vi "Check_Traverse_move.vi"(0 "Current position":sgl[](array[numeric])=[0.0, 0.0, 0.0] format="%.2f", 1 "Traverse Name":string, 2 "Full Check":bool, 5 "New Position":sgl[](array[numeric])=[0.0, 0.0, 0.0] format="%.2f", 7 "Model       Roll      Pitch       Yaw (deg)":sgl[](array[numeric]) format="%#.2f", 9 "Probe Volume":T1=[{"Max"=15.0, "Min"=-15.0}, {"Max"=250.0, "Min"=0.0}, {"Max"=15.0, "Min"=-15.0}] {"Min" format="%#.1f"; "Max" format="%#.1f"}, 11 "Entire Space":T1=[{"Max"=15001.0, "Min"=12000.0}, {"Max"=1000.0, "Min"=-1000.0}, {"Max"=700.0, "Min"=0.0}] {"Min" format="%#.1f"; "Max" format="%#.1f"}, 12 "Exclude Array":T2[](array[typedef])=[{"Sizes"=[{"Max"=15000.0, "Min"=0.0}, {"Max"=1000.0, "Min"=-1000.0}, {"Max"=300.0, "Min"=0.0}], "Name"="Roughness Elements", "Exclude Type"=enum."Allow only vertical moves"}, {"Sizes"=[{"Max"=17000.0, "Min"=16000.0}, {"Max"=200.0, "Min"=-200.0}, {"Max"=-50.0, "Min"=-250.0}], "Name"="B204", "Exclude Type"=enum."Exclude completely"}] {"Sizes"."Min" format="%#.1f"; "Sizes"."Max" format="%#.1f"}, 13 "Probe Support":T1=[{"Max"=15001.0, "Min"=12000.0}, {"Max"=1000.0, "Min"=-1000.0}, {"Max"=700.0, "Min"=0.0}] {"Min" format="%#.1f"; "Max" format="%#.1f"}) -> (6 "Position At Crash":dbl[](array[numeric]) format="%.2f", 10 "Steps":sgl[][](array[numeric]) format="%.2f", 15 "Error Comments":string)   [LabVIEW 2020]
uses:
  Box_size.ctl
  Exclude_cluster.ctl
  Exclusion_type.ctl
panel:
  # "X                Y                   Z"
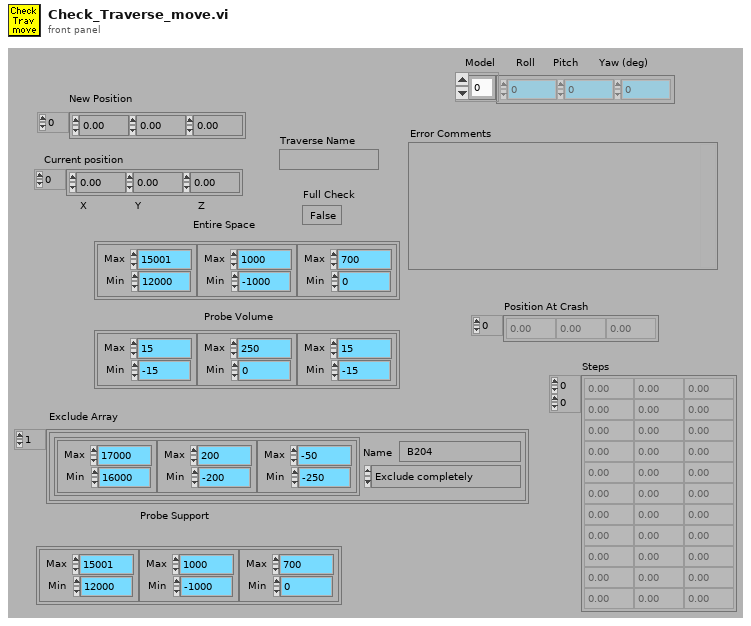
[diagram p1: front panel]
types:
  T1 = typedef "Box_size.ctl" = cluster{"Max":sgl, "Min":sgl}[]
  T2 = typedef "Exclude_cluster.ctl" = cluster{"Sizes":T1, "Name":string, "Exclude Type":T3}
  T3 = typedef "Exclusion_type.ctl" = enum16{"Exclude completely", "Allow only vertical moves"}
  T4 = enum16{"To Traverse Coordinates", "To User Coordinates"}
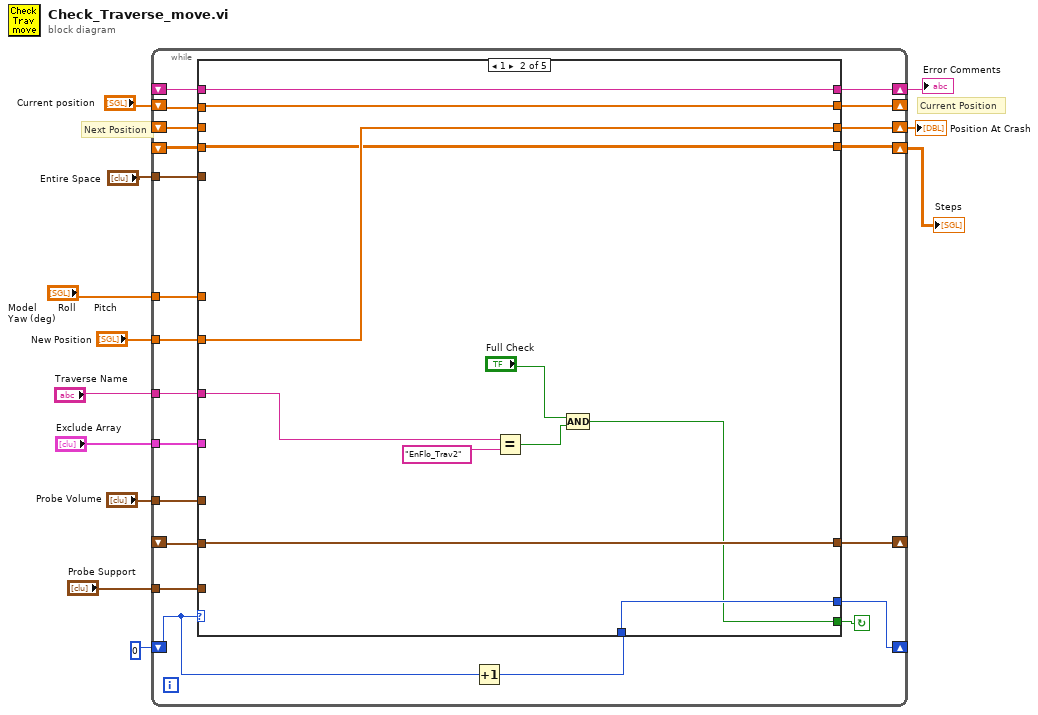
[diagram p0: block diagram]
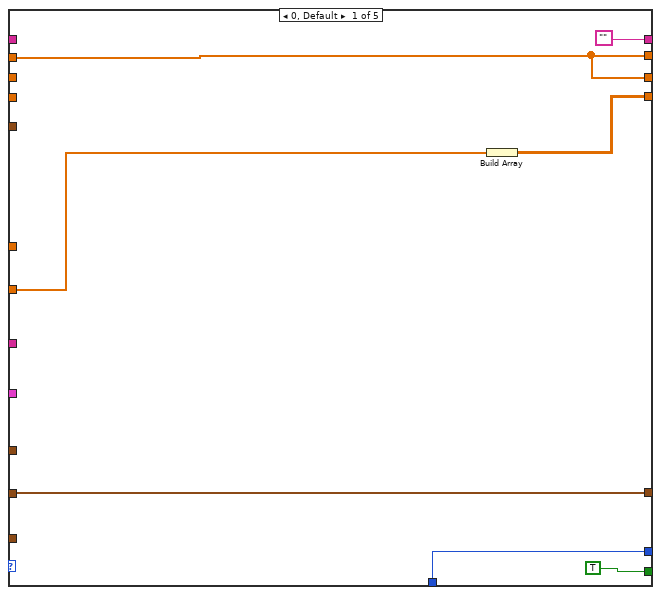
[diagram p2: hidden frame]
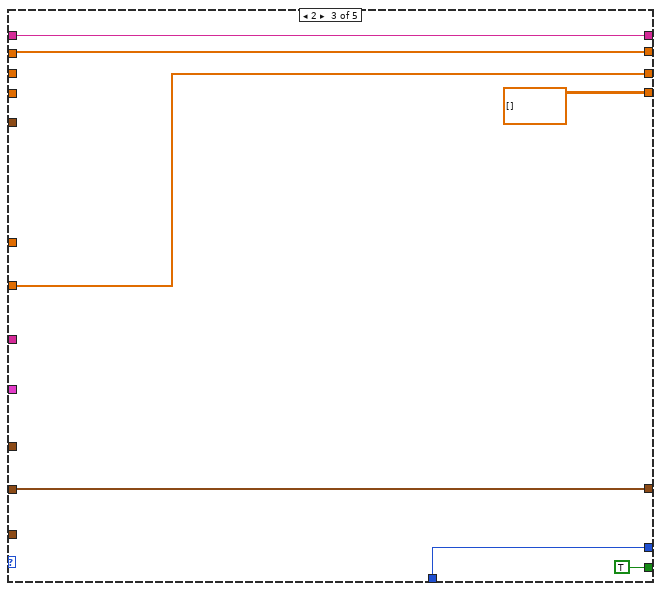
[diagram p3: hidden frame]
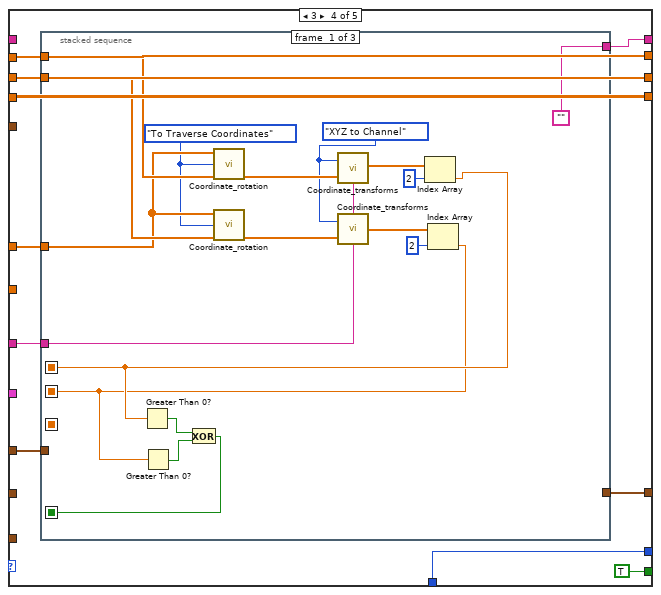
[diagram p4: hidden frame]
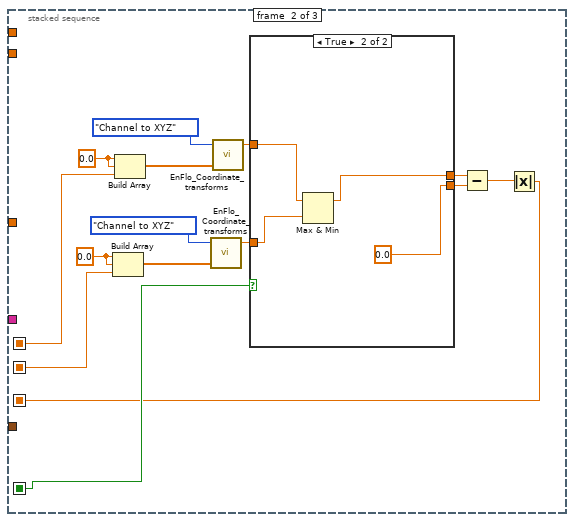
[diagram p5: hidden frame]
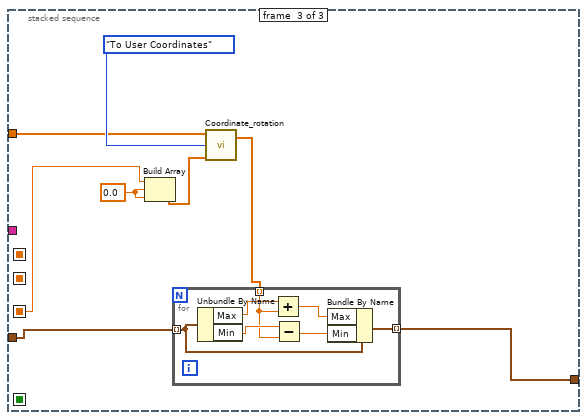
[diagram p7: hidden frame]
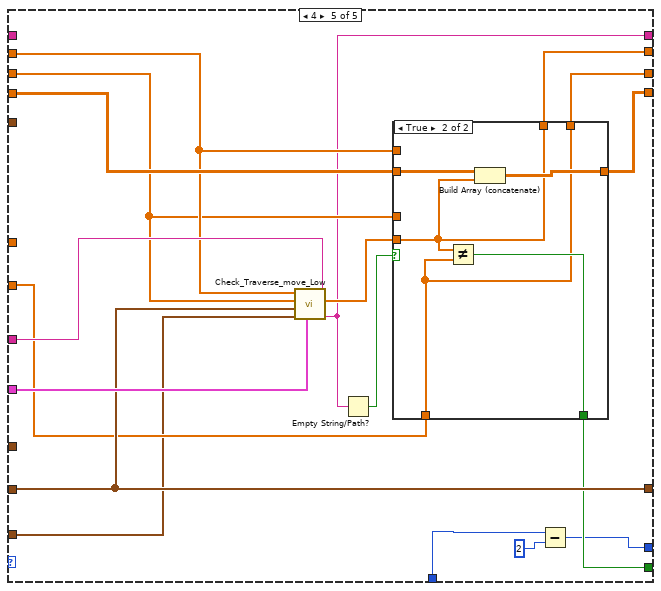
[diagram p8: hidden frame]
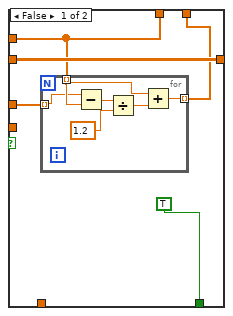
[diagram p9: hidden frame]
diagram:
  # "Current Position"
  # "Next Position"
  n1 = while {
    shift-left: _ -> [w15]
    shift-right: [w14] -> w3
    tunnel: "Probe Volume" -> [w16]
    shift-left: _ -> [w18]
    shift-right: [w17] -> _
    tunnel: "Model       Roll      Pitch       Yaw (deg)" -> [w19]
    tunnel: "New Position" -> [w20]
    shift-left: _ -> [w22]
    shift-right: [w23] -> w7
    shift-left: 0 -> [w26]
    shift-right: [w25] -> _
    tunnel: "Traverse Name" -> [w27]
    tunnel: "Entire Space" -> [w28]
    tunnel: "Exclude Array" -> [w29]
    shift-left: _ -> [w21]
    shift-right: [w31] -> w5
    shift-left: "Current position" -> [w33]
    shift-right: [w32] -> _
    tunnel: "Probe Support" -> [w13]
    stop <- w30 continue-if-true
    n2 = Increment(x=w26) -> (x+1=w24:i32)
    n3 = case shown="1" w26 {
      tunnel: w33 -> [w34 w50 w57 w65 w126]
      tunnel: [w34 w50 w57 w65 w131] -> w32
      tunnel: [w34 w43 w54 w64 w130] -> w31
      tunnel: [TRUE ("Box Inside") w45 TRUE ("Box Inside") TRUE ("Box Inside") w133] -> w30
      tunnel: w18 -> [w40 w49 w56 _ w138]
      tunnel: w29 -> [_ _ _ _ w140]
      tunnel: w28 -> [_ _ _ _ _]
      tunnel: w27 -> [_ w46 _ w62 w139]
      tunnel: [w36 w48 w55 w60 w128] -> w25
      tunnel: w24 -> [w36 w48 w55 w60 w127]
      tunnel: ["" w51 w58 w68 w123] -> w23
      tunnel: w22 -> [_ w51 w58 _ _]
      tunnel: w21 -> [_ _ _ w64 w125]
      tunnel: w20 -> [w39 w43 w54 _ w134]
      tunnel: w19 -> [_ _ _ w63 _]
      tunnel: [w40 w49 w56 w66 w138] -> w17
      tunnel: w16 -> [_ _ _ w61 _]
      tunnel: w15 -> [_ w42 _ w59 w137]
      tunnel: [w38 w42 dbl[][] [] w59 w136] -> w14
      tunnel: w13 -> [_ _ _ _ w124]
      frame 0, Default {
        n4 = Build Array(w39) -> (w38:sgl[][])
      }
      frame 1 {
        n5 = Equal?(x=w46, y="EnFlo_Trav2") -> (x = y?=w41:bool)
        n6 = Compound Arithmetic op=AND("Full Check", w41) -> (w45:bool)
      }
      frame 2 {
      }
      frame 3 {
        n7 = stacked-sequence {
          seq-local: [w71 _ _] -> [_ w101 _]
          seq-local: [w70 _ _] -> [_ w100 _]
          seq-local: [w69 _ _] -> [_ w91 _]
          seq-local: [_ w87 _] -> [_ _ w110]
          tunnel: ["" _ _] -> w68
          tunnel: [_ _ w114] -> w66
          tunnel: w65 -> [w84 _ _]
          tunnel: w64 -> [w82 _ _]
          tunnel: w63 -> [w81 _ w108]
          tunnel: w62 -> [w80 _ _]
          tunnel: w61 -> [_ _ w115]
          frame #0 {
            w78 = enum16{"XYZ to Channel", "Channel to XYZ"}."XYZ to Channel" ("Mode")
            w79 = T4."To Traverse Coordinates" ("Mode")
            n8 = call "Coordinate_rotation.vi"("Roll-Pitch-Yaw"=w81, "Input Position"=w84, "Mode"=w79) -> ("Output Position"=w85:sgl[])  [unwired: 2 in, 1 out]
            n9 = call "Coordinate_rotation.vi"("Roll-Pitch-Yaw"=w81, "Input Position"=w82, "Mode"=w79) -> ("Output Position"=w83:sgl[])  [unwired: 2 in, 1 out]
            n10 = call "Coordinate_transforms.vi"("Traverse Name"=w80, "Input"=w85, "Mode"=w78) -> ("Output"=w77:sgl[])
            n11 = call "Coordinate_transforms.vi"("Traverse Name"=w80, "Input"=w83, "Mode"=w78) -> ("Output"=w74:sgl[])
            n12 = Index Array(array=w77, index=2) -> (element=w71:sgl)
            n13 = Greater Than 0?(x=w71) -> (x > 0?=w73:bool)
            n14 = Index Array(array=w74, index=2) -> (element=w70:sgl)
            n15 = Greater Than 0?(x=w70) -> (x > 0?=w72:bool)
            n16 = Exclusive Or(1:w72, 2:w73) -> (0:w69:bool)
          }
          frame #1 {
            w94 = 0.0 ("element")
            w99 = 0.0 ("element")
            n17 = Build Array(w94, w94, w100) -> (w96:dbl[])
            n18 = Build Array(w99, w99, w101) -> (w97:dbl[])
            n19 = call "EnFlo_Coordinate_transforms.vi"("Input"=w96, "Mode"=enum16{"XYZ to Channel", "Channel to XYZ"}."Channel to XYZ") -> ("X theta"=w92:dbl)  [unwired: 3 out]
            n20 = call "EnFlo_Coordinate_transforms.vi"("Input"=w97, "Mode"=enum16{"XYZ to Channel", "Channel to XYZ"}."Channel to XYZ") -> ("X theta"=w93:dbl)  [unwired: 3 out]
            n21 = case shown="True" w91 {
              tunnel: w93 -> [w103 w106]
              tunnel: w92 -> [w102 w107]
              tunnel: [w102 0.0 ("element")] -> w90
              tunnel: [w103 w105] -> w89
              frame False {
              }
              frame True {
                n22 = Max & Min(x=w106, y=w107) -> (max(x,y)=w105:dbl)  [unwired: 1 out]
              }
            }
            n23 = Subtract(x=w89, y=w90) -> (x-y=w88:dbl)
            n24 = Absolute Value(x=w88) -> (abs(x)=w87:dbl)
          }
          frame #2 {
            w112 = 0.0 ("Input Element")
            n25 = Build Array(w110, w112, w112) -> (w111:dbl[])
            n26 = call "Coordinate_rotation.vi"("Roll-Pitch-Yaw"=w108, "Input Position"=w111, "Mode"=T4."To User Coordinates") -> ("Output Position"=w109:sgl[])  [unwired: 2 in, 1 out]
            n27 = for {
              tunnel: w115 -> [w122] mode=indexing
              tunnel: w109 -> [w117] mode=indexing
              tunnel: [w116] -> w114 mode=indexing
              n28 = Unbundle By Name(w122) -> ("Max"=w121:sgl, "Min"=w120:sgl)
              n29 = Add(x=w121, y=w117) -> (x+y=w119:sgl)
              n30 = Subtract(x=w120, y=w117) -> (x-y=w118:sgl)
              n31 = Bundle By Name(cluster=w122, "Max"=w119, "Min"=w118) -> (w116:cluster{"Max":sgl, "Min":sgl})
            }
          }
        }
      }
      frame 4 {
        n32 = call "Check_Traverse_move_Low.vi"("Traverse Name"=w139, "Exclude Array"=w140, "Probe Support"=w124, "Probe Volume"=w138, "New Position"=w125, "Current position"=w126) -> ("Error Comments"=w123:string, "Position At Crash"=w132:dbl[])  [unwired: 1 in, 1 out]
        n33 = Empty String/Path?(string/path=w123) -> (empty?=w135:bool)
        n34 = case shown="True" w135 {
          tunnel: w137 -> [w145 w156]
          tunnel: w132 -> [_ w153]
          tunnel: [w145 w155] -> w136
          tunnel: w134 -> [_ w152]
          tunnel: [TRUE w154] -> w133
          tunnel: [w143 w153] -> w131
          tunnel: [w141 w152] -> w130
          tunnel: w126 -> [w143 _]
          tunnel: w125 -> [w142 _]
          frame False {
            n35 = for {
              tunnel: w143 -> [w147] mode=indexing
              tunnel: w142 -> [w146] mode=indexing
              tunnel: [w148] -> w141 mode=indexing
              n36 = Subtract(x=w146, y=w147) -> (x-y=w151:dbl)
              n37 = Divide(x=w151, y=1.2) -> (x/y=w149:dbl)
              n38 = Add(x=w147, y=w149) -> (x+y=w148:dbl)
            }
          }
          frame True {
            n39 = Not Equal?(x=w153, y=w152) -> (x != y?=w154:bool)
            n40 = Build Array (concatenate)(w156, w153) -> (w155:dbl[][])
          }
        }
        n41 = Subtract(x=w127, y=2) -> (x-y=w128:i32)
      }
    }
  }
  "Error Comments" <- w7
  "Position At Crash" <- w5
  "Steps" <- w3
